vi "magnetotropic -- V3.vi"(0 "B":dbl[](array[numeric])=[3.7119054620880973e-32, 0.0, 9.9], 1 "n":dbl[](array[numeric])=[1.0, 0.0, 6.123233995736766e-17], 2 "g":dbl[](array[numeric])=[1.0, 1.0, 2.0], 3 "JR":dbl, 4 "JO":dbl, 5 "JK":dbl, 7 "G":dbl[](array[numeric])=[1.0, 1.0, 2.0], 8 "spins":enum16{"spin one half", "bipartite"}(ring), 9 "nsteps":i32=100, 11 "temperature":dbl(slide)=1.0 scale=0.0..100.0) -> (14 "magnetotropic":dbl=15.765581836122678)   [LabVIEW 2018]
uses:
  <vilib>/Analysis/Matrix/Datatypes/ComplexMatrix.ctl
  <vilib>/Analysis/7linalg.llb/Complex Matrix Exp.vi
  <vilib>/Analysis/baseanly.llb/Complex A x B.vi
  <vilib>/Analysis/_algsub.llb/Complex Matrix Trace.vi
  <vilib>/imath/engines/lvmath2/RunTimeEngine/IndexRead/NIMS V(S).vi
  <instcachedir>/0/NIMS V(S)_0488751826AF41519A22953C041130DC.lvgen/NIMS V(S)_0488751826AF41519A22953C041130DC_000.vi
  <vilib>/imath/engines/lvmath2/RunTimeEngine/ErrorHandling/NIMS_Create Error From Enums.vi
  <vilib>/Analysis/Matrix/Numeric/Conversions/Array To Matrix - CA2.vi
  <vilib>/imath/engines/lvmath2/RunTimeEngine/NodeEndStatement/NIMS_NodeEndStatement_Output.vi
  <instcachedir>/0/NIMS_NodeEndStatement_Output_53EC0D466D134D7ABD903AC30B43404B.lvgen/NIMS_NodeEndStatement_Output_53EC0D466D134D7ABD903AC30B43404B_009.vi
  <vilib>/imath/engines/lvmath2/RunTimeEngine/ErrorHandling/NIMS_Finalize Error.vi
  <vilib>/Analysis/Matrix/Numeric/Multiply/Multiply - CM,C.vi
  <vilib>/Analysis/NI_AALBase.lvlib
  <vilib>/Analysis/NI_AALPro.lvlib
  <vilib>/Analysis/Matrix/NI_Matrix.lvlib
panel:
  out "H0":T1=[[19.8+0.0i, 3.7119054620880973e-32+0.0i], [3.7119054620880973e-32+0.0i, -19.8+0.0i]] caption="Complex Matrix"
  out "dadaH":T1=[[-19.8+0.0i, 6.062001655779399e-16+0.0i], [6.062001655779399e-16+0.0i, 19.8+0.0i]] caption="Complex Matrix"
  out "daH":T1=[[0.0+0.0i, 0.0+9.9i], [0.0-9.9i, 0.0+0.0i]] caption="Complex Matrix"
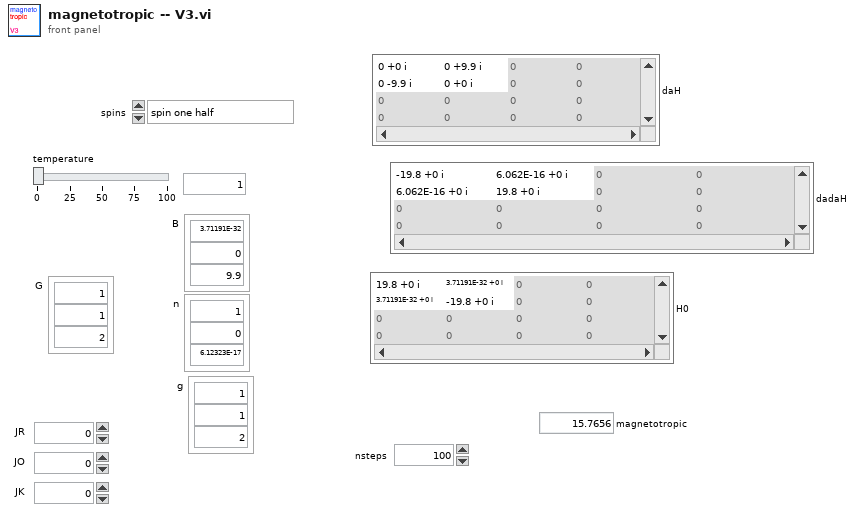
[diagram p1: front panel]
types:
  T1 = typedef "NI_Matrix.lvlib/ComplexMatrix.ctl" = cdb[][]
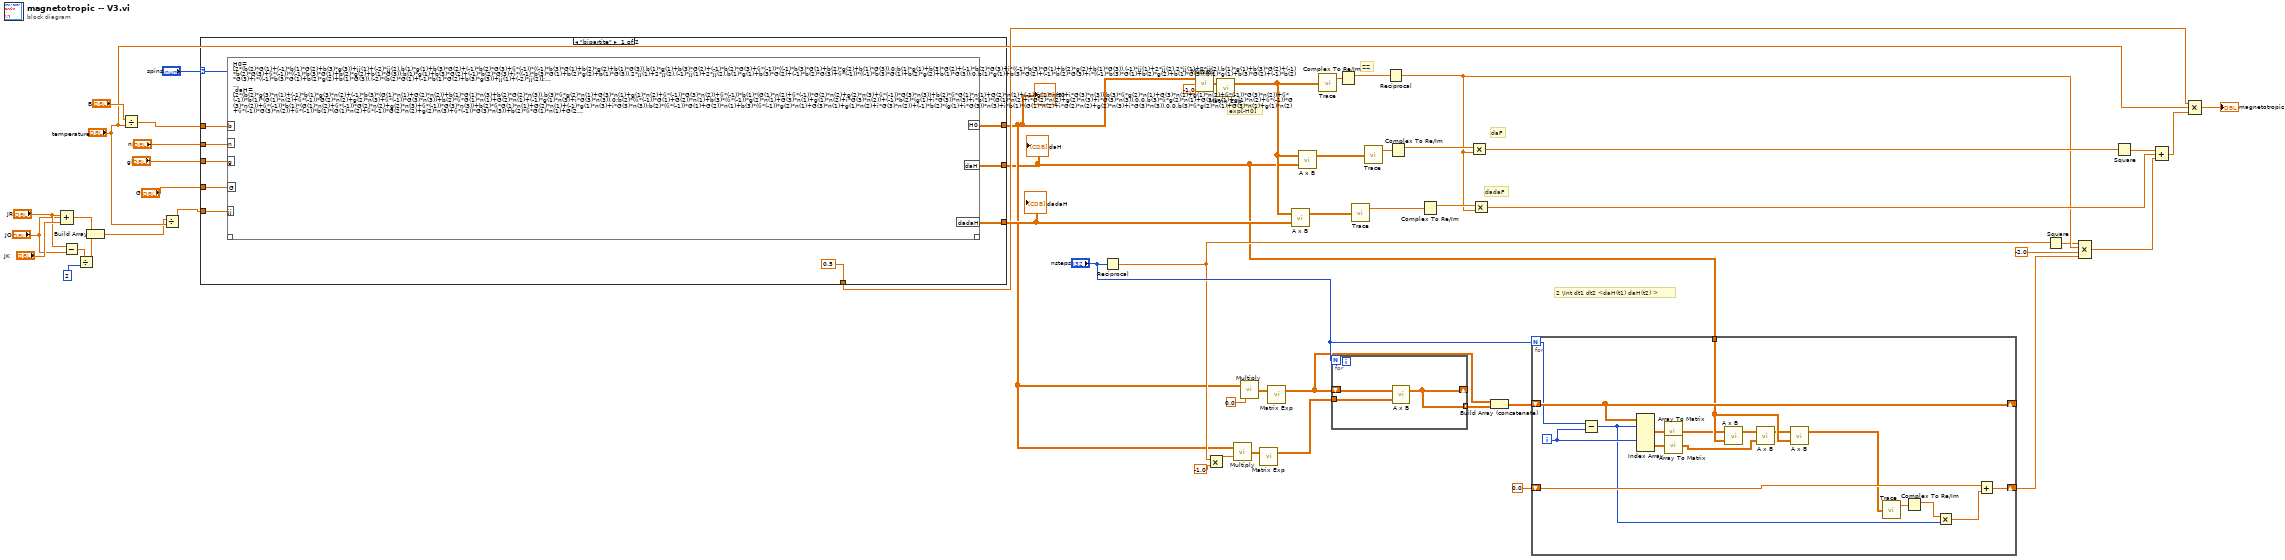
[diagram p0: block diagram]
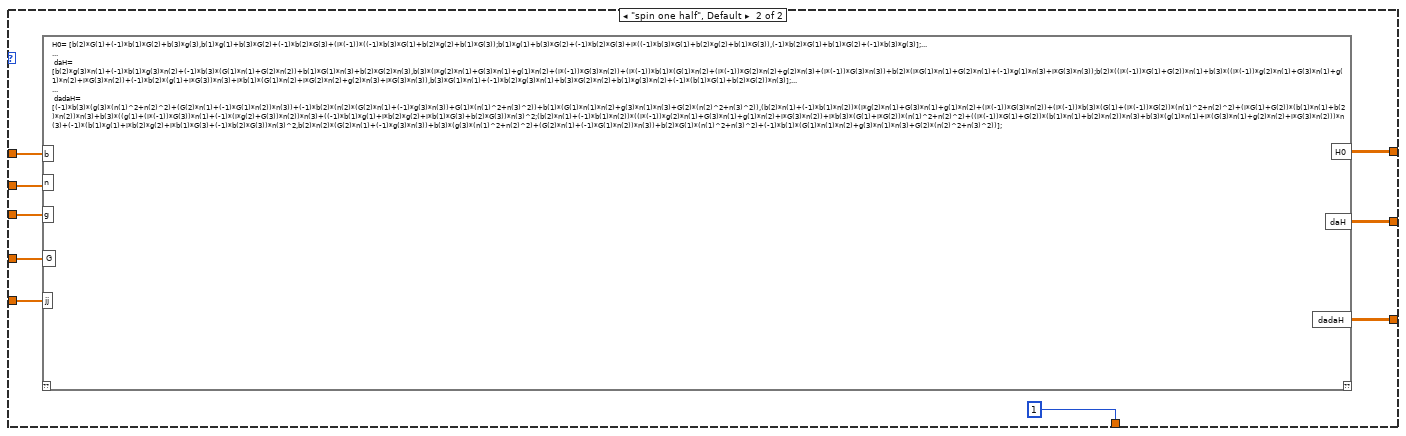
[diagram p2: hidden frame]
diagram:
  # "2 \\Int dt1 dt2 <daH(t1) daH(t2) >"
  # "dadaF"
  # "daF"
  # "exp[-H0]"
  # "ZZ"
  n1 = Compound Arithmetic op=ADD("JR", "JO", "JK") -> (w8:dbl)
  n2 = Subtract(x="JR", y="JO") -> (x-y=w5:dbl)
  n3 = Divide(x=w5, y=2) -> (x/y=w3:dbl)
  n4 = Build Array(w8, w3) -> (w2:dbl[])
  n5 = Divide(x="B", y="temperature") -> (x/y=w27:dbl[])
  n6 = Divide(x=w2, y="temperature") -> (x/y=w26:dbl[])
  n7 = case shown="\"bipartite\"" "spins" {
    tunnel: w27 -> [w62 w4569]
    tunnel: "n" -> [w61 w4568]
    tunnel: "g" -> [w60 w4567]
    tunnel: w26 -> [w59 w4566]
    tunnel: [w58 w4565] -> w15
    tunnel: [w57 w4564] -> w10
    tunnel: [w56 w4563] -> w36
    tunnel: [0.5 1] -> w24
    tunnel: "G" -> [w54 w4561]
    frame "bipartite" {
      n8 = mathscript code="H0= [2*(b(2)*G(1)+(-1)*b(1)*G(2)+b(3)*g(3))+jj(1)+(-2)*jj(2),b(1)*g(1)+b(3)*G(2)+(-1)*b(2)*G(3)+(i*(-1))*((-1)*b(3)*G(1)+b(2)*g(2)+b(1)*G(3)),b(1)*g(1)+b(3)*G(2)+(-1)*b(2)*G(3)+(i*(-1))*((-1)*b(3)*G(1)+b(2)*g(2)+b(1)*G(3)),0;b(1)*g(1)+b(3)*G(2)+(-1)*b(2)*G(3)+i*((-1)*b(3)*G(1)+b(2)*g(2)+b(1)*G(3)),(-1)*jj(1)+2*jj(2),2*jj(1)+2*jj(2),b(1)*g(1)+b(3)*G(2)+(-1)*b(2)*G(3)+(i*(-1))*((-1)*b(3)*G(1)+b(2)*g(2)+b(1)*G(3));b(1)*g(1)+b(3)*G(2)+(-1)*b(2)*G(3)+i*((-1)*b(3)*G(1)+b(2)*g(2)+b(1)*G(3)),2*jj(1)+2*jj(2),(-1)*jj(1)+2*jj(2),b(1)*g(1)+b(3)*G(2)+(-1)*b(2)*G(3)+(i*(-1))*((-1)*b(3)*G(1)+b(2)*g(2)+b(1)*G(3));0,b(1)*g(1)+b(3)*G(2)+(-1)*b(2)*G(3)+i*((-1)*b(3)*G(1)+b(2)*g(2)+b(1)*G(3)),b(1)*g(1)+b(3)*G(2)+(-1)*b(2)*G(3)+i*((-1)*b(3)*G(1)+b(2)*g(2)+b(1)*G(3)),(-2)*(b(2)*G(1)+(-1)*b(1)*G(2)+b(3)*g(3))+jj(1)+(-2)*jj(2)];...\n...\n daH= [2*(b(2)*g(3)*n(1)+(-1)*b(1)*g(3)*n(2)+(-1)*b(3)*(G(1)*n(1)+G(2)*n(2))+b(1)*G(1)*n(3)+b(2)*G(2)*n(3)),b(3)*(i*g(2)*n(1)+G(3)*n(1)+g(1)*n(2)+(i*(-1))*G(3)*n(2))+(i*(-1))*b(1)*(G(1)*n(2)+(i*(-1))*G(2)*n(2)+g(2)*n(3)+(i*(-1))*G(3)*n(3))+b(2)*(i*G(1)*n(1)+G(2)*n(1)+(-1)*g(1)*n(3)+i*G(3)*n(3)),b(3)*(i*g(2)*n(1)+G(3)*n(1)+g(1)*n(2)+(i*(-1))*G(3)*n(2))+(i*(-1))*b(1)*(G(1)*n(2)+(i*(-1))*G(2)*n(2)+g(2)*n(3)+(i*(-1))*G(3)*n(3))+b(2)*(i*G(1)*n(1)+G(2)*n(1)+(-1)*g(1)*n(3)+i*G(3)*n(3)),0;b(2)*((i*(-1))*G(1)+G(2))*n(1)+b(3)*((i*(-1))*g(2)*n(1)+G(3)*n(1)+g(1)*n(2)+i*G(3)*n(2))+(-1)*b(2)*(g(1)+i*G(3))*n(3)+i*b(1)*(G(1)*n(2)+i*G(2)*n(2)+g(2)*n(3)+i*G(3)*n(3)),0,0,b(3)*(i*g(2)*n(1)+G(3)*n(1)+g(1)*n(2)+(i*(-1))*G(3)*n(2))+(i*(-1))*b(1)*(G(1)*n(2)+(i*(-1))*G(2)*n(2)+g(2)*n(3)+(i*(-1))*G(3)*n(3))+b(2)*(i*G(1)*n(1)+G(2)*n(1)+(-1)*g(1)*n(3)+i*G(3)*n(3));b(2)*((i*(-1))*G(1)+G(2))*n(1)+b(3)*((i*(-1))*g(2)*n(1)+G(3)*n(1)+g(1)*n(2)+i*G(3)*n(2))+(-1)*b(2)*(g(1)+i*G(3))*n(3)+i*b(1)*(G(1)*n(2)+i*G(2)*n(2)+g(2)*n(3)+i*G(3)*n(3)),0,0,b(3)*(i*g(2)*n(1)+G(3)*n(1)+g(1)*n(2)+(i*(-1))*G(3)*n(2))+(i*(-1))*b(1)*(G(1)*n(2)+(i*(-1))*G(2)*n(2)+g(2)*n(3)+(i*(-1))*G(3)*n(3))+b(2)*(i*G(1)*n(1)+G(2)*n(1)+(-1)*g(1)*n(3)+i*G(3)*n(3));0,b(2)*((i*(-1))*G(1)+G(2))*n(1)+b(3)*((i*(-1))*g(2)*n(1)+G(3)*n(1)+g(1)*n(2)+i*G(3)*n(2))+(-1)*b(2)*(g(1)+i*G(3))*n(3)+i*b(1)*(G(1)*n(2)+i*G(2)*n(2)+g(2)*n(3)+i*G(3)*n(3)),b(2)*((i*(-1))*G(1)+G(2))*n(1)+b(3)*((i*(-1))*g(2)*n(1)+G(3)*n(1)+g(1)*n(2)+i*G(3)*n(2))+(-1)*b(2)*(g(1)+i*G(3))*n(3)+i*b(1)*(G(1)*n(2)+i*G(2)*n(2)+g(2)*n(3)+i*G(3)*n(3)),(-2)*(b(2)*g(3)*n(1)+(-1)*b(1)*g(3)*n(2)+(-1)*b(3)*(G(1)*n(1)+G(2)*n(2))+b(1)*G(1)*n(3)+b(2)*G(2)*n(3))];...\n...\n dadaH= [(-2)*b(3)*(g(3)*(n(1)^2+n(2)^2)+(G(2)*n(1)+(-1)*G(1)*n(2))*n(3))+(-2)*b(2)*(n(2)*(G(2)*n(1)+(-1)*g(3)*n(3))+G(1)*(n(1)^2+n(3)^2))+2*b(1)*(G(1)*n(1)*n(2)+g(3)*n(1)*n(3)+G(2)*(n(2)^2+n(3)^2)),(b(2)*n(1)+(-1)*b(1)*n(2))*(i*g(2)*n(1)+G(3)*n(1)+g(1)*n(2)+(i*(-1))*G(3)*n(2))+(i*(-1))*b(3)*(G(1)+(i*(-1))*G(2))*(n(1)^2+n(2)^2)+(i*G(1)+G(2))*(b(1)*n(1)+b(2)*n(2))*n(3)+b(3)*((g(1)+(i*(-1))*G(3))*n(1)+(-1)*(i*g(2)+G(3))*n(2))*n(3)+((-1)*b(1)*g(1)+i*b(2)*g(2)+i*b(1)*G(3)+b(2)*G(3))*n(3)^2,(b(2)*n(1)+(-1)*b(1)*n(2))*(i*g(2)*n(1)+G(3)*n(1)+g(1)*n(2)+(i*(-1))*G(3)*n(2))+(i*(-1))*b(3)*(G(1)+(i*(-1))*G(2))*(n(1)^2+n(2)^2)+(i*G(1)+G(2))*(b(1)*n(1)+b(2)*n(2))*n(3)+b(3)*((g(1)+(i*(-1))*G(3))*n(1)+(-1)*(i*g(2)+G(3))*n(2))*n(3)+((-1)*b(1)*g(1)+i*b(2)*g(2)+i*b(1)*G(3)+b(2)*G(3))*n(3)^2,0;(b(2)*n(1)+(-1)*b(1)*n(2))*((i*(-1))*g(2)*n(1)+G(3)*n(1)+g(1)*n(2)+i*G(3)*n(2))+i*b(3)*(G(1)+i*G(2))*(n(1)^2+n(2)^2)+((i*(-1))*G(1)+G(2))*(b(1)*n(1)+b(2)*n(2))*n(3)+b(3)*(g(1)*n(1)+i*(G(3)*n(1)+g(2)*n(2)+i*G(3)*n(2)))*n(3)+(-1)*(b(1)*g(1)+i*b(2)*g(2)+i*b(1)*G(3)+(-1)*b(2)*G(3))*n(3)^2,0,0,(b(2)*n(1)+(-1)*b(1)*n(2))*(i*g(2)*n(1)+G(3)*n(1)+g(1)*n(2)+(i*(-1))*G(3)*n(2))+(i*(-1))*b(3)*(G(1)+(i*(-1))*G(2))*(n(1)^2+n(2)^2)+(i*G(1)+G(2))*(b(1)*n(1)+b(2)*n(2))*n(3)+b(3)*((g(1)+(i*(-1))*G(3))*n(1)+(-1)*(i*g(2)+G(3))*n(2))*n(3)+((-1)*b(1)*g(1)+i*b(2)*g(2)+i*b(1)*G(3)+b(2)*G(3))*n(3)^2;(b(2)*n(1)+(-1)*b(1)*n(2))*((i*(-1))*g(2)*n(1)+G(3)*n(1)+g(1)*n(2)+i*G(3)*n(2))+i*b(3)*(G(1)+i*G(2))*(n(1)^2+n(2)^2)+((i*(-1))*G(1)+G(2))*(b(1)*n(1)+b(2)*n(2))*n(3)+b(3)*(g(1)*n(1)+i*(G(3)*n(1)+g(2)*n(2)+i*G(3)*n(2)))*n(3)+(-1)*(b(1)*g(1)+i*b(2)*g(2)+i*b(1)*G(3)+(-1)*b(2)*G(3))*n(3)^2,0,0,(b(2)*n(1)+(-1)*b(1)*n(2))*(i*g(2)*n(1)+G(3)*n(1)+g(1)*n(2)+(i*(-1))*G(3)*n(2))+(i*(-1))*b(3)*(G(1)+(i*(-1))*G(2))*(n(1)^2+n(2)^2)+(i*G(1)+G(2))*(b(1)*n(1)+b(2)*n(2))*n(3)+b(3)*((g(1)+(i*(-1))*G(3))*n(1)+(-1)*(i*g(2)+G(3))*n(2))*n(3)+((-1)*b(1)*g(1)+i*b(2)*g(2)+i*b(1)*G(3)+b(2)*G(3))*n(3)^2;0,(b(2)*n(1)+(-1)*b(1)*n(2))*((i*(-1))*g(2)*n(1)+G(3)*n(1)+g(1)*n(2)+i*G(3)*n(2))+i*b(3)*(G(1)+i*G(2))*(n(1)^2+n(2)^2)+((i*(-1))*G(1)+G(2))*(b(1)*n(1)+b(2)*n(2))*n(3)+b(3)*(g(1)*n(1)+i*(G(3)*n(1)+g(2)*n(2)+i*G(3)*n(2)))*n(3)+(-1)*(b(1)*g(1)+i*b(2)*g(2)+i*b(1)*G(3)+(-1)*b(2)*G(3))*n(3)^2,(b(2)*n(1)+(-1)*b(1)*n(2))*((i*(-1))*g(2)*n(1)+G(3)*n(1)+g(1)*n(2)+i*G(3)*n(2))+i*b(3)*(G(1)+i*G(2))*(n(1)^2+n(2)^2)+((i*(-1))*G(1)+G(2))*(b(1)*n(1)+b(2)*n(2))*n(3)+b(3)*(g(1)*n(1)+i*(G(3)*n(1)+g(2)*n(2)+i*G(3)*n(2)))*n(3)+(-1)*(b(1)*g(1)+i*b(2)*g(2)+i*b(1)*G(3)+(-1)*b(2)*G(3))*n(3)^2,2*b(3)*(g(3)*(n(1)^2+n(2)^2)+(G(2)*n(1)+(-1)*G(1)*n(2))*n(3))+2*b(2)*(n(2)*(G(2)*n(1)+(-1)*g(3)*n(3))+G(1)*(n(1)^2+n(3)^2))+(-2)*b(1)*(G(1)*n(1)*n(2)+g(3)*n(1)*n(3)+G(2)*(n(2)^2+n(3)^2))];..."("b"=w62, "n"=w61, "g"=w60, "jj"=w59, "G"=w54) -> ("H0"=w58:T1, "daH"=w57:T1, "dadaH"=w56:T1)  [unwired: 1 in, 1 out]
    }
    frame "spin one half", Default {
      n9 = mathscript code="H0= [b(2)*G(1)+(-1)*b(1)*G(2)+b(3)*g(3),b(1)*g(1)+b(3)*G(2)+(-1)*b(2)*G(3)+(i*(-1))*((-1)*b(3)*G(1)+b(2)*g(2)+b(1)*G(3));b(1)*g(1)+b(3)*G(2)+(-1)*b(2)*G(3)+i*((-1)*b(3)*G(1)+b(2)*g(2)+b(1)*G(3)),(-1)*b(2)*G(1)+b(1)*G(2)+(-1)*b(3)*g(3)];...\n...\n daH= [b(2)*g(3)*n(1)+(-1)*b(1)*g(3)*n(2)+(-1)*b(3)*(G(1)*n(1)+G(2)*n(2))+b(1)*G(1)*n(3)+b(2)*G(2)*n(3),b(3)*(i*g(2)*n(1)+G(3)*n(1)+g(1)*n(2)+(i*(-1))*G(3)*n(2))+(i*(-1))*b(1)*(G(1)*n(2)+(i*(-1))*G(2)*n(2)+g(2)*n(3)+(i*(-1))*G(3)*n(3))+b(2)*(i*G(1)*n(1)+G(2)*n(1)+(-1)*g(1)*n(3)+i*G(3)*n(3));b(2)*((i*(-1))*G(1)+G(2))*n(1)+b(3)*((i*(-1))*g(2)*n(1)+G(3)*n(1)+g(1)*n(2)+i*G(3)*n(2))+(-1)*b(2)*(g(1)+i*G(3))*n(3)+i*b(1)*(G(1)*n(2)+i*G(2)*n(2)+g(2)*n(3)+i*G(3)*n(3)),b(3)*G(1)*n(1)+(-1)*b(2)*g(3)*n(1)+b(3)*G(2)*n(2)+b(1)*g(3)*n(2)+(-1)*(b(1)*G(1)+b(2)*G(2))*n(3)];...\n...\n dadaH= [(-1)*b(3)*(g(3)*(n(1)^2+n(2)^2)+(G(2)*n(1)+(-1)*G(1)*n(2))*n(3))+(-1)*b(2)*(n(2)*(G(2)*n(1)+(-1)*g(3)*n(3))+G(1)*(n(1)^2+n(3)^2))+b(1)*(G(1)*n(1)*n(2)+g(3)*n(1)*n(3)+G(2)*(n(2)^2+n(3)^2)),(b(2)*n(1)+(-1)*b(1)*n(2))*(i*g(2)*n(1)+G(3)*n(1)+g(1)*n(2)+(i*(-1))*G(3)*n(2))+(i*(-1))*b(3)*(G(1)+(i*(-1))*G(2))*(n(1)^2+n(2)^2)+(i*G(1)+G(2))*(b(1)*n(1)+b(2)*n(2))*n(3)+b(3)*((g(1)+(i*(-1))*G(3))*n(1)+(-1)*(i*g(2)+G(3))*n(2))*n(3)+((-1)*b(1)*g(1)+i*b(2)*g(2)+i*b(1)*G(3)+b(2)*G(3))*n(3)^2;(b(2)*n(1)+(-1)*b(1)*n(2))*((i*(-1))*g(2)*n(1)+G(3)*n(1)+g(1)*n(2)+i*G(3)*n(2))+i*b(3)*(G(1)+i*G(2))*(n(1)^2+n(2)^2)+((i*(-1))*G(1)+G(2))*(b(1)*n(1)+b(2)*n(2))*n(3)+b(3)*(g(1)*n(1)+i*(G(3)*n(1)+g(2)*n(2)+i*G(3)*n(2)))*n(3)+(-1)*(b(1)*g(1)+i*b(2)*g(2)+i*b(1)*G(3)+(-1)*b(2)*G(3))*n(3)^2,b(2)*n(2)*(G(2)*n(1)+(-1)*g(3)*n(3))+b(3)*(g(3)*(n(1)^2+n(2)^2)+(G(2)*n(1)+(-1)*G(1)*n(2))*n(3))+b(2)*G(1)*(n(1)^2+n(3)^2)+(-1)*b(1)*(G(1)*n(1)*n(2)+g(3)*n(1)*n(3)+G(2)*(n(2)^2+n(3)^2))];"("b"=w4569, "n"=w4568, "g"=w4567, "jj"=w4566, "G"=w4561) -> ("H0"=w4565:T1, "daH"=w4564:T1, "dadaH"=w4563:T1)  [unwired: 1 in, 1 out]
    }
  }
  "daH" <- w10
  "dadaH" <- w36
  "H0" <- w15
  n10 = Reciprocal(x="nsteps") -> (1/x=w20:dbl)
  n11 = call-poly <vilib>:"Multiply.vi"("Complex Scalar c"=-1.0, "Complex Matrix A"=w15) -> ("A * c"=w50:T1)
  n12 = Multiply(x=w20, y=-1.0) -> (x*y=w19:dbl)
  n13 = call-poly <vilib>:"Matrix Exp.vi"("Input Matrix"=w50) -> ("Matrix Exp"=w35:T1)  [unwired: 1 in, 1 out]
  n14 = call-poly <vilib>:"Multiply.vi"("Complex Scalar c"=w19, "Complex Matrix A"=w15) -> ("A * c"=w18:T1)
  n15 = call-poly <vilib>:"Multiply.vi"("Complex Scalar c"=0.0, "Complex Matrix A"=w15) -> ("A * c"=w16:T1)
  n16 = call-poly <vilib>:"Matrix Exp.vi"("Input Matrix"=w18) -> ("Matrix Exp"=w17:T1)  [unwired: 1 in, 1 out]
  n17 = call-poly <vilib>:"Matrix Exp.vi"("Input Matrix"=w16) -> ("Matrix Exp"=w12:T1)  [unwired: 1 in, 1 out]
  n18 = call-poly <vilib>:"A x B.vi"("B"=w36, "A"=w35) -> ("A x B"=w45:T1)  [unwired: 1 out]
  n19 = call-poly <vilib>:"A x B.vi"("B"=w10, "A"=w35) -> ("A x B"=w49:T1)  [unwired: 1 out]
  n20 = call-poly <vilib>:"Trace.vi"("Input Matrix"=w35) -> ("trace"=w47:cdb)  [unwired: 1 out]
  n21 = for {
    N: "nsteps" -> [_]
    tunnel: w17 -> [w6159]
    shift-right: [w6158] -> _
    shift-left: w12 -> [w6160]
    tunnel: [w6158] -> w13 mode=indexing
    n22 = call-poly <vilib>:"A x B.vi"("B"=w6159, "A"=w6160) -> ("A x B"=w6158:T1)  [unwired: 1 out]
  }
  n23 = Complex To Re/Im(x + iy=w47) -> (x=w40:dbl)  [unwired: 1 out]
  n24 = call-poly <vilib>:"Trace.vi"("Input Matrix"=w45) -> ("trace"=w44:cdb)  [unwired: 1 out]
  n25 = call-poly <vilib>:"Trace.vi"("Input Matrix"=w49) -> ("trace"=w48:cdb)  [unwired: 1 out]
  n26 = Reciprocal(x=w40) -> (1/x=w32:dbl)
  n27 = Complex To Re/Im(x + iy=w48) -> (x=w46:dbl)  [unwired: 1 out]
  n28 = Complex To Re/Im(x + iy=w44) -> (x=w43:dbl)  [unwired: 1 out]
  n29 = Multiply(x=w46, y=w32) -> (x*y=w39:dbl)
  n30 = Multiply(x=w43, y=w32) -> (x*y=w37:dbl)
  n31 = Build Array (concatenate)(w12, w13) -> (w11:cdb[][][])
  n32 = for {
    N: "nsteps" -> [w6174]
    shift-right: [w6175] -> w30
    shift-left: 0.0 -> [w6176]
    shift-right: [w6177] -> _
    shift-left: w11 -> [w6177]
    tunnel: w10 -> [w6173]
    i -> [w6164]
    n33 = Subtract(x=w6174, y=w6164) -> (x-y=w6162:i32)
    n34 = Index Array(array=w6177, index (dim 0) #1=w6162, index (dim 0) #2=w6164) -> (element #1=w6169:cdb[][], element #2=w6170:cdb[][])  [unwired: 4 in]
    n35 = call-poly <vilib>:"Array To Matrix.vi"("Complex 2D Array"=w6169) -> ("Complex Matrix"=w6168:T1)
    n36 = call-poly <vilib>:"Array To Matrix.vi"("Complex 2D Array"=w6170) -> ("Complex Matrix"=w6167:T1)
    n37 = call-poly <vilib>:"A x B.vi"("B"=w6173, "A"=w6168) -> ("A x B"=w6172:T1)  [unwired: 1 out]
    n38 = call-poly <vilib>:"A x B.vi"("B"=w6167, "A"=w6172) -> ("A x B"=w6166:T1)  [unwired: 1 out]
    n39 = call-poly <vilib>:"A x B.vi"("B"=w6173, "A"=w6166) -> ("A x B"=w6163:T1)  [unwired: 1 out]
    n40 = call-poly <vilib>:"Trace.vi"("Input Matrix"=w6163) -> ("trace"=w6171:cdb)  [unwired: 1 out]
    n41 = Complex To Re/Im(x + iy=w6171) -> (x=w6165:dbl)  [unwired: 1 out]
    n42 = Multiply(x=w6165, y=w6162) -> (x*y=w6161:dbl)
    n43 = Add(x=w6176, y=w6161) -> (x+y=w6175:dbl)
  }
  n44 = Square(x=w20) -> (x^2=w29:dbl)
  n45 = Compound Arithmetic op=MULTIPLY(w29, w32, -2.0 ("y"), w30) -> (w31:dbl)
  n46 = Square(x=w39) -> (x^2=w38:dbl)
  n47 = Compound Arithmetic op=ADD(w38, w37, w31) -> (w23:dbl)
  n48 = Compound Arithmetic op=MULTIPLY(w24, "temperature", w23) -> (→"magnetotropic":dbl)
